vi "set temp.vi"(8 "error in (no error)":errorcluster caption="Fehler (Eingang, kein Fehler)", 10 "temp":string, 11 "Norm (Eingang)":refnum<class "Norm.lvclass">) -> (0 "error out":errorcluster caption="Fehler (Ausgang)", 3 "Norm (Ausgang)":refnum<class "Norm.lvclass">)   [LabVIEW 2013, in "DatenKlassen.lvlib" / "Norm.lvclass"]
uses:
  Norm.lvclass
  Norm.lvclass/Norm.ctl
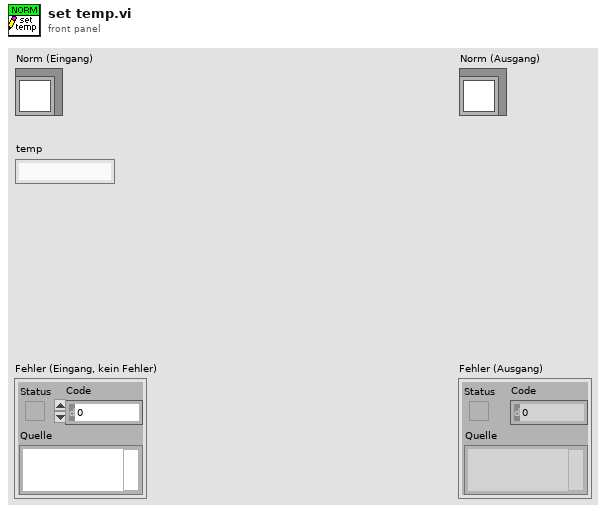
[diagram p1: front panel]
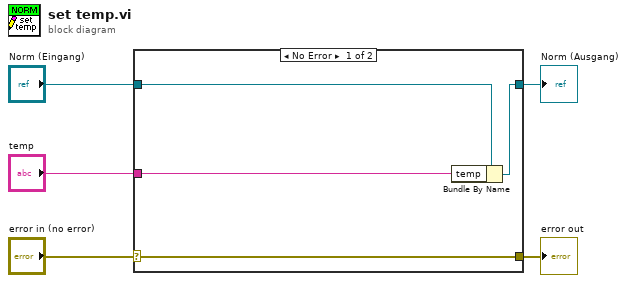
[diagram p0: block diagram]
diagram:
  n1 = case shown="No Error" "error in (no error)" {
    selector: "error in (no error)" -> [w9 w10]
    tunnel: [w9 w10] -> w4
    tunnel: [w7 w11] -> w2
    tunnel: "Norm (Eingang)" -> [w8 w11]
    tunnel: "temp" -> [w6 _]
    frame No Error {
      n2 = Bundle By Name(cluster=w8, "temp"=w6) -> (w7:refnum<class "Norm.lvclass">)
    }
    frame Error {
    }
  }
  "error out" <- w4
  "Norm (Ausgang)" <- w2
